vi "ScanProgramState.vi"(11 "programState in":string) -> (3 "programState out":T1)   [LabVIEW 2016, in "Universal Robot.lvclass"]
uses:
  Universal Robot.lvclass
  ProgramState.ctl
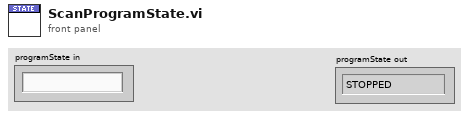
[diagram p1: front panel]
types:
  T1 = typedef "Universal Robot.lvclass/ProgramState.ctl" = enum16{"STOPPED", "PLAYING", "PAUSE"}
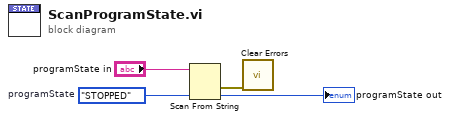
[diagram p0: block diagram]
diagram:
  w2 = ProgramState."STOPPED"  # programState
  n1 = Scan From String(input string="programState in", default 1=w2) -> (error out=w3:errorcluster, output 1=→"programState out":T1)  [unwired: 3 in, 2 out]
  n2 = call <vilib>:"Clear Errors.vi"("error in (no error)"=w3) -> ()  [unwired: 5 in, 2 out]
